vi "ScanDCSOpticalSwitch.vi"(0 "Optical Output":T1, 1 "DAQ Port":tag, 2 "Time Left (ms)":refnum<vi>, 3 "Update Time (ms):":refnum<vi>, 4 "Duration Time (ms):":refnum<vi>, 5 "Detectors Select":enum32{"4 Detectors", "8 Detectors"}(ring), 6 "Optical Input":T2, 7 "Detector\n Buttons":refnum<vi>, 8 "Number of Scans":i32, 9 "Detector Indicator":refnum<vi>, 10 "File Path:":path, 11 "g2":refnum<vi>, 12 "File Name:":string, 13 "Computer time":refnum<vi>, 14 "X index":i32, 15 "Y index":i32) -> ()   [LabVIEW 2011]
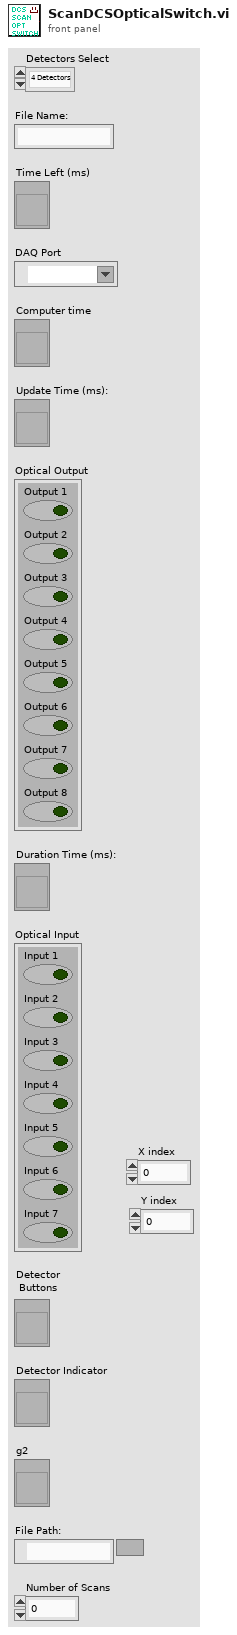
[diagram p1: front panel]
types:
  T1 = cluster{"Output 1":bool, "Output 2":bool, "Output 3":bool, "Output 4":bool, "Output 5":bool, "Output 6":bool, "Output 7":bool, "Output 8":bool}
  T2 = cluster{"Input 1":bool, "Input 2":bool, "Input 3":bool, "Input 4":bool, "Input 5":bool, "Input 6":bool, "Input 7":bool}
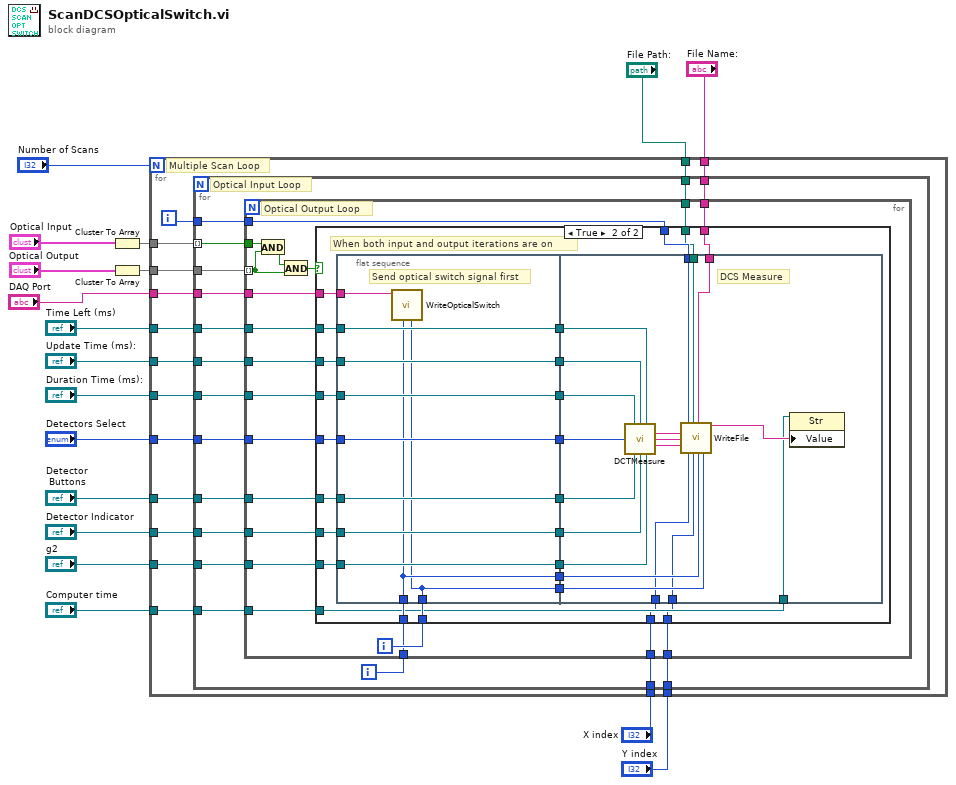
[diagram p0: block diagram]
diagram:
  n1 = Cluster To Array(cluster="Optical Input") -> (array=w15:bool[])
  n2 = Cluster To Array(cluster="Optical Output") -> (array=w13:bool[])
  n3 = for {
    N: "Number of Scans" -> [_]
    tunnel: "File Path:" -> [w34]
    tunnel: "File Name:" -> [w33]
    tunnel: "g2" -> [w32]
    tunnel: "Detector Indicator" -> [w31]
    tunnel: "Detector\n Buttons" -> [w30]
    tunnel: "Detectors Select" -> [w29]
    tunnel: "Duration Time (ms):" -> [w28]
    tunnel: "Update Time (ms):" -> [w27]
    tunnel: "Time Left (ms)" -> [w26]
    tunnel: w13 -> [w25]
    tunnel: w15 -> [w24]
    tunnel: "DAQ Port" -> [w22]
    tunnel: "Computer time" -> [w21]
    tunnel: "X index" -> [w20]
    tunnel: "Y index" -> [w19]
    i -> [w23]
    # "Multiple Scan Loop"
    n4 = for {
      tunnel: w24 -> [w50] mode=indexing
      tunnel: w25 -> [w51]
      tunnel: w26 -> [w49]
      tunnel: w27 -> [w48]
      tunnel: w28 -> [w47]
      tunnel: w29 -> [w46]
      tunnel: w30 -> [w45]
      tunnel: w31 -> [w44]
      tunnel: w32 -> [w43]
      tunnel: w33 -> [w41]
      tunnel: w34 -> [w40]
      tunnel: w23 -> [w39]
      tunnel: w22 -> [w38]
      tunnel: w21 -> [w37]
      tunnel: w20 -> [w36]
      tunnel: w19 -> [w35]
      i -> [w42]
      # "Optical Input Loop"
      n5 = for {
        tunnel: w51 -> [w69] mode=indexing
        tunnel: w50 -> [w71]
        tunnel: w49 -> [w67]
        tunnel: w48 -> [w66]
        tunnel: w47 -> [w65]
        tunnel: w46 -> [w64]
        tunnel: w45 -> [w63]
        tunnel: w44 -> [w62]
        tunnel: w43 -> [w61]
        tunnel: w42 -> [w59]
        tunnel: w41 -> [w58]
        tunnel: w40 -> [w57]
        tunnel: w39 -> [w56]
        tunnel: w38 -> [w55]
        tunnel: w37 -> [w54]
        tunnel: w36 -> [w53]
        tunnel: w35 -> [w52]
        i -> [w60]
        # "Optical Output Loop"
        n6 = And(x=w71, y=w69) -> (x .and. y?=w70:bool)
        n7 = And(x=w70, y=w69) -> (x .and. y?=w68:bool)
        n8 = case shown="True" w68 {
          tunnel: w67 -> [_ w92]
          tunnel: w66 -> [_ w90]
          tunnel: w65 -> [_ w88]
          tunnel: w64 -> [_ w86]
          tunnel: w63 -> [_ w84]
          tunnel: w62 -> [_ w82]
          tunnel: w61 -> [_ w80]
          tunnel: w60 -> [_ w94]
          tunnel: w59 -> [_ w95]
          tunnel: w58 -> [_ w78]
          tunnel: w57 -> [_ w77]
          tunnel: w56 -> [_ w79]
          tunnel: w55 -> [_ w96]
          tunnel: w54 -> [_ w74]
          tunnel: w53 -> [_ w73]
          tunnel: w52 -> [_ w72]
          frame False {
            # "Do nothing\n\nAlone..... alone.......aloooone"
          }
          frame True {
            # "When both input and output iterations are on"
            n9 = flat-sequence {
              tunnel: w96 -> [w106]
              tunnel: w95 -> [w98]
              tunnel: w94 -> [w97]
              tunnel: [w105] -> w93
              tunnel: w92 -> [w105]
              tunnel: [w104] -> w91
              tunnel: w90 -> [w104]
              tunnel: [w103] -> w89
              tunnel: w88 -> [w103]
              tunnel: [w102] -> w87
              tunnel: w86 -> [w102]
              tunnel: [w101] -> w85
              tunnel: w84 -> [w101]
              tunnel: [w100] -> w83
              tunnel: w82 -> [w100]
              tunnel: [w99] -> w81
              tunnel: w80 -> [w99]
              tunnel: [w98] -> w76
              tunnel: [w97] -> w75
              tunnel: w93 -> [w117]
              tunnel: w91 -> [w116]
              tunnel: w89 -> [w115]
              tunnel: w87 -> [w121]
              tunnel: w85 -> [w114]
              tunnel: w83 -> [w113]
              tunnel: w81 -> [w112]
              tunnel: w79 -> [w120]
              tunnel: w78 -> [w119]
              tunnel: w77 -> [w118]
              tunnel: w76 -> [w111]
              tunnel: w75 -> [w110]
              tunnel: w74 -> [w109]
              tunnel: w73 -> [w108]
              tunnel: w72 -> [w107]
              frame #0 {
                # "Send optical switch signal first"
                n10 = call "WriteOpticalSwitch.vi"("Output"=w97, "Input"=w98, "DAQ Port"=w106) -> ()  [unwired: 9 in]
              }
              frame #1 {
                # "DCS Measure"
                n11 = call "DCTMeasure.vi"("Duration Time"=w115, "Update Time"=w116, "Time Left"=w117, "Detectors Select"=w121, "Detector Buttons"=w114, "Detector Indicators"=w113, "g2"=w112) -> ("Intensity data"=w124:string, "tau data"=w123:string, "g2 data"=w122:string)  [unwired: 6 in]
                n12 = call "WriteFile.vi"("Intensity data"=w124, "Tau data"=w123, "g2 data"=w122, "Scan"=w120, "X Index"=w108, "Data Save Directory:"=w118, "Y Index"=w107, "File Name:"=w119, "Optical Input"=w111, "Optical Output"=w110) -> ("Computer Time"=w125:string)  [unwired: 8 in, 1 out]
                n13 = property class="Str"(reference=w109, "Value"=w125) -> ()  [unwired: 1 in, 2 out]
              }
            }
          }
        }
      }
    }
  }
